vi "New from TCP.vi"(7 "From":refnum<class "Endpoint.lvclass">, 10 "TCP Connection":refnum<k5>, 11 "URI":refnum<class "URI.lvclass">) -> (0 "error out":errorcluster, 3 "Client":refnum<class "Websocket Client.lvclass">)   [LabVIEW 2020, in "Stream-Websocket.lvlib" / "Websocket Client.lvclass"]
uses:
  Websocket Client.lvclass
  lv-stream/stream/URI/URI.lvclass
  lv-stream/stream/Endpoint/Endpoint.lvclass
  C:/dev/lv20CE/relink/lv-stream/stream/Endpoint/Endpoint.lvclass
  C:/dev/lv20CE/relink/lv-stream/stream/Connection/Connection.lvclass
  Websocket Client.lvclass/Websocket Client.ctl
  lv-stream/stream/Connection State.ctl
  lv-stream/stream/Connection/State.ctl
  lv-stream/stream/Stream.lvlib
  lv-stream/stream/Connection/Connection.lvclass
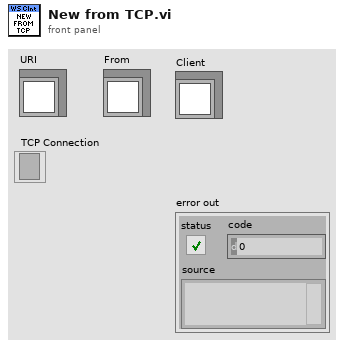
[diagram p1: front panel]
types:
  T1 = typedef "Stream.lvlib/Connection.lvclass/State.ctl" = enum16{"Closed", "Idle", "Connecting", "Connected", "Shutdown"}
  T2 = typedef "Stream.lvlib/Connection State.ctl" = enum16{"Connected", "Disconnected"}
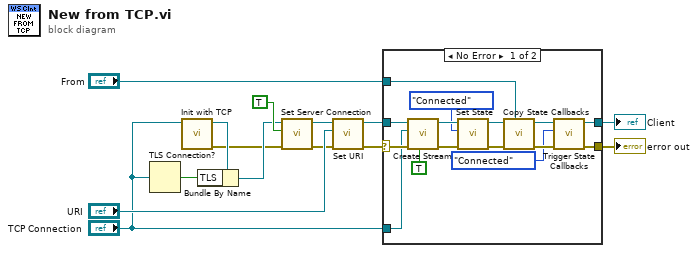
[diagram p0: block diagram]
diagram:
  n1 = TLS Connection?(1:"TCP Connection") -> (0:w2:bool)
  n2 = call "Init with TCP.vi"("TCP Connection"="TCP Connection") -> ("error out"=w5:errorcluster, "Websocket Client out"=w6:refnum<class "Websocket Client.lvclass">)  [unwired: 9 in]
  n3 = Bundle By Name(cluster=w6, "TLS"=w2) -> (w7:refnum<class "Websocket Client.lvclass">)
  n4 = call "Set Server Connection.vi"("error in (no error)"=w5, "Server Connection"=TRUE, "Websocket Client in"=w7) -> ("error out"=w3:errorcluster, "Websocket Client out"=w4:refnum<class "Websocket Client.lvclass">)  [unwired: 7 in]
  n5 = call "Set URI.vi"("error in (no error)"=w3, "URI"="URI", "Endpoint in"=w4) -> ("error out"=w10:errorcluster, "Endpoint out"=w9:refnum<class "Websocket Client.lvclass">)  [unwired: 7 in]
  n6 = case shown="No Error" w10 {
    selector: w10 -> [w28 w30]
    tunnel: w9 -> [w29 w31]
    tunnel: "TCP Connection" -> [w27 _]
    tunnel: "From" -> [w19 _]
    tunnel: [w18 w31] -> w12
    tunnel: [w17 w30] -> w11
    frame No Error {
      n7 = call "Create Stream.vi"("Server Stream"=TRUE, "error in (no error)"=w28, "TCP Connection"=w27, "Websocket Client in"=w29) -> ("error out"=w20:errorcluster, "Websocket Client out"=w21:refnum<class "Websocket Client.lvclass">)  [unwired: 6 in]
      n8 = call "Set State.vi"("error in (no error)"=w20, "State"=State."Connected", "Connection in"=w21) -> ("error out"=w23:errorcluster, "Connection out"=w22:refnum<class "Websocket Client.lvclass">)  [unwired: 7 in]
      n9 = call "Copy State Callbacks.vi"("From"=w19, "error in (no error)"=w23, "Endpoint in"=w22) -> ("error out"=w25:errorcluster, "Endpoint out"=w26:refnum<class "Websocket Client.lvclass">)  [unwired: 7 in]
      n10 = call "Trigger State Callbacks.vi"("error in (no error)"=w25, "State"=Connection_State."Connected", "Connection in"=w26) -> ("error out"=w17:errorcluster, "Connection out"=w18:refnum<class "Websocket Client.lvclass">)  [unwired: 7 in]
    }
    frame Error {
    }
  }
  "Client" <- w12
  "error out" <- w11
